vi "Generate Firmware Wizard Summary Message.vi"(8 "Error In":errorcluster, 10 "Device ID":u8, 11 "Device Family":T1 items=["National Instruments", "Digilent", "Arduino"]) -> (0 "Error Out":errorcluster, 3 "Summary":string)   [LabVIEW 2011, in "LVH-LINX.lvlib"]
uses:
  LVH-LINX.lvlib
  Type Defs/Device Family.ctl
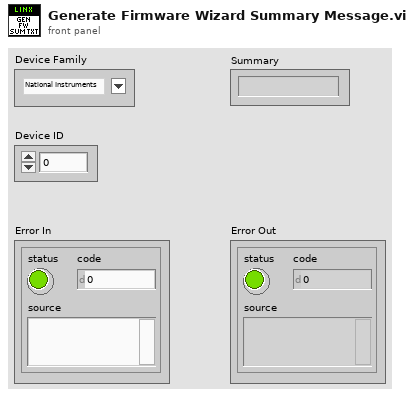
[diagram p1: front panel]
types:
  T1 = typedef "LVH-LINX.lvlib/Device Family.ctl" = u16
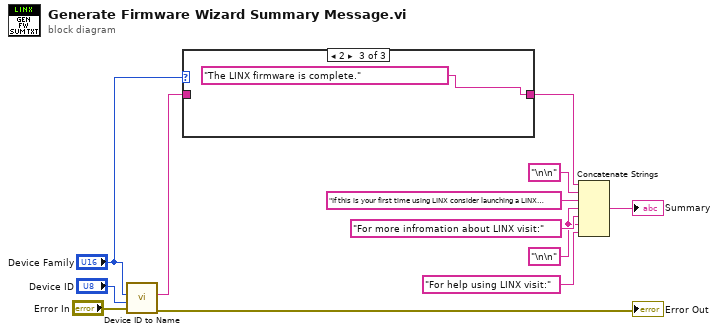
[diagram p0: block diagram]
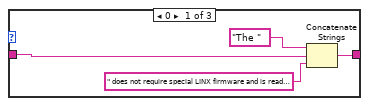
[diagram p2: hidden frame]
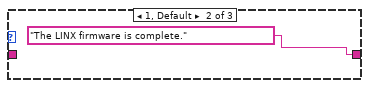
[diagram p3: hidden frame]
diagram:
  w5 = "\n\n" ("string")
  n1 = call "Device ID to Name.vi"("Error In"="Error In", "Device Index"="Device ID", "Family Index"="Device Family") -> ("Error Out"=→"Error Out":errorcluster, "Device Name"=w1:string)  [unwired: 6 in, 1 out]
  n2 = case shown="2" "Device Family" {
    tunnel: [w14 "The LINX firmware is complete." "The LINX firmware is complete."] -> w3
    tunnel: w1 -> [w13 _ _]
    frame 0 {
      n3 = Concatenate Strings("The ", w13, " does not require special LINX firmware and is ready to use." ("string")) -> (w14:string)
    }
    frame 1, Default {
    }
    frame 2 {
    }
  }
  n4 = Concatenate Strings(w3, "\n\n" ("string"), "If this is your first time using LINX consider launching a LINX example using the button below.  More LINX examples can befound in the LabVIEW Example Finder by launching LabVIEW and clicking Help>>Find Examples, then searching for 'LINX'." ("string"), w5, "For more infromation about LINX visit:" ("string"), w5, "For help using LINX visit:" ("string")) -> (→"Summary":string)
